vi "AttackerStop.vi"(6 "atacando contra?":bool, 7 "AI Parameters":T1={"GotoKick"={"Dist do cone a frente"=150.0, "attacker farback"=1500.0, "Perto"=300.0, "Dist a frente da bola"=0.0, "min dist to kick"=150.0, "Constante do Renault"=0.05, "distance between ball and robot"=200.0, "Time Target \nto transition"=0.3}, "Attacker"={"CC chute"=0.09, "CC passe"=0.045, "Kick Force"=100.0}, "Defender"={"D max"=1700.0, "Velocidade p/ o robô avançar"=1000.0, "Kick Force"=100.0}, "Timeout"={"Field/v in x"=6, "Dist Robots"=300, "Dist up in y"=300}, "Pose Striker"={"dist"=200.0, "Numeric"=-4.0, "dist 2"=200.0}, "Dist Stop"=300.0, "Distance when ball out"=200, "Defence central gap "=150.0} {"Defence central gap" format="%#_13g"; "Dist Stop" format="%#_13g"; "Pose Striker"."Numeric" format="%#_13g"; "Defender"."Kick Force" format="%#_13g"; "Defender"."Velocidade p/ o robô avançar" format="%#_13g"; "Attacker"."Kick Force" format="%#_13g"; "Attacker"."CC passe" format="%#_13g"; "Attacker"."CC chute" format="%#_13g"; "GotoKick"."distance between ball and robot" format="%#_13g"; "GotoKick"."min dist to kick" format="%#_13g"; "GotoKick"."Dist a frente da bola" format="%#_13g"; "GotoKick"."Perto" format="%#_13g"; "GotoKick"."attacker farback" format="%#_13g"; "GotoKick"."Dist do cone a frente" format="%#_13g"}, 8 "IA State Input 2":T2, 9 "balls":T6[](array[typedef]), 10 "Field Size in":T7, 11 "Robot in":T3={"id"=0, "function"=enum."Attacker", "x"=0.0, "y"=0.0, "orientation"=0.0, "v_tangent"=0.0, "v_normal"=0.0, "v_ang"=0.0, "kick_x"=0.0, "kick_z"=0.0, "dribble"=FALSE, "Timestamp"=timestamp(0 s since 1904-01-01), "dest_x"=0.0, "dest_y"=0.0, "dest_orientation"=0.0, "estimatives"={"est_v_tangent"=0.0, "est_v_normal"=0.0, "est_vx"=0.0, "est_vy"=0.0, "Pos Robot Est"=[]}, "dest_x_kick"=0.0, "dest_y_kick"=0.0, "Gap Coord"=[], "States"=enum."GoToTangent"}) -> (3 "Robot out":T3={"id"=0, "function"=enum."Attacker", "x"=0.0, "y"=0.0, "orientation"=0.0, "v_tangent"=0.0, "v_normal"=0.0, "v_ang"=0.0, "kick_x"=0.0, "kick_z"=0.0, "dribble"=FALSE, "Timestamp"=timestamp(0 s since 1904-01-01), "dest_x"=0.0, "dest_y"=0.0, "dest_orientation"=0.0, "estimatives"={"est_v_tangent"=0.0, "est_v_normal"=0.0, "est_vx"=0.0, "est_vy"=0.0, "Pos Robot Est"=[]}, "dest_x_kick"=0.0, "dest_y_kick"=0.0, "Gap Coord"=[], "States"=enum."GoToTangent"})   [LabVIEW 2016]
uses:
  Core/Field Size.ctl
  Core/AI Robot.ctl
  Functions Enum.ctl
  AttackerStates.ctl
  Core/AI Ball.ctl
  Core/AI Input.ctl
  Core/AI Judge.ctl
  Command Enum.ctl
  Util/Events/Events.ctl
  AI Parameters.ctl
  <vilib>/Analysis/_algsub.llb/Real Vector Norm.vi
  <vilib>/Analysis/NI_AALPro.lvlib
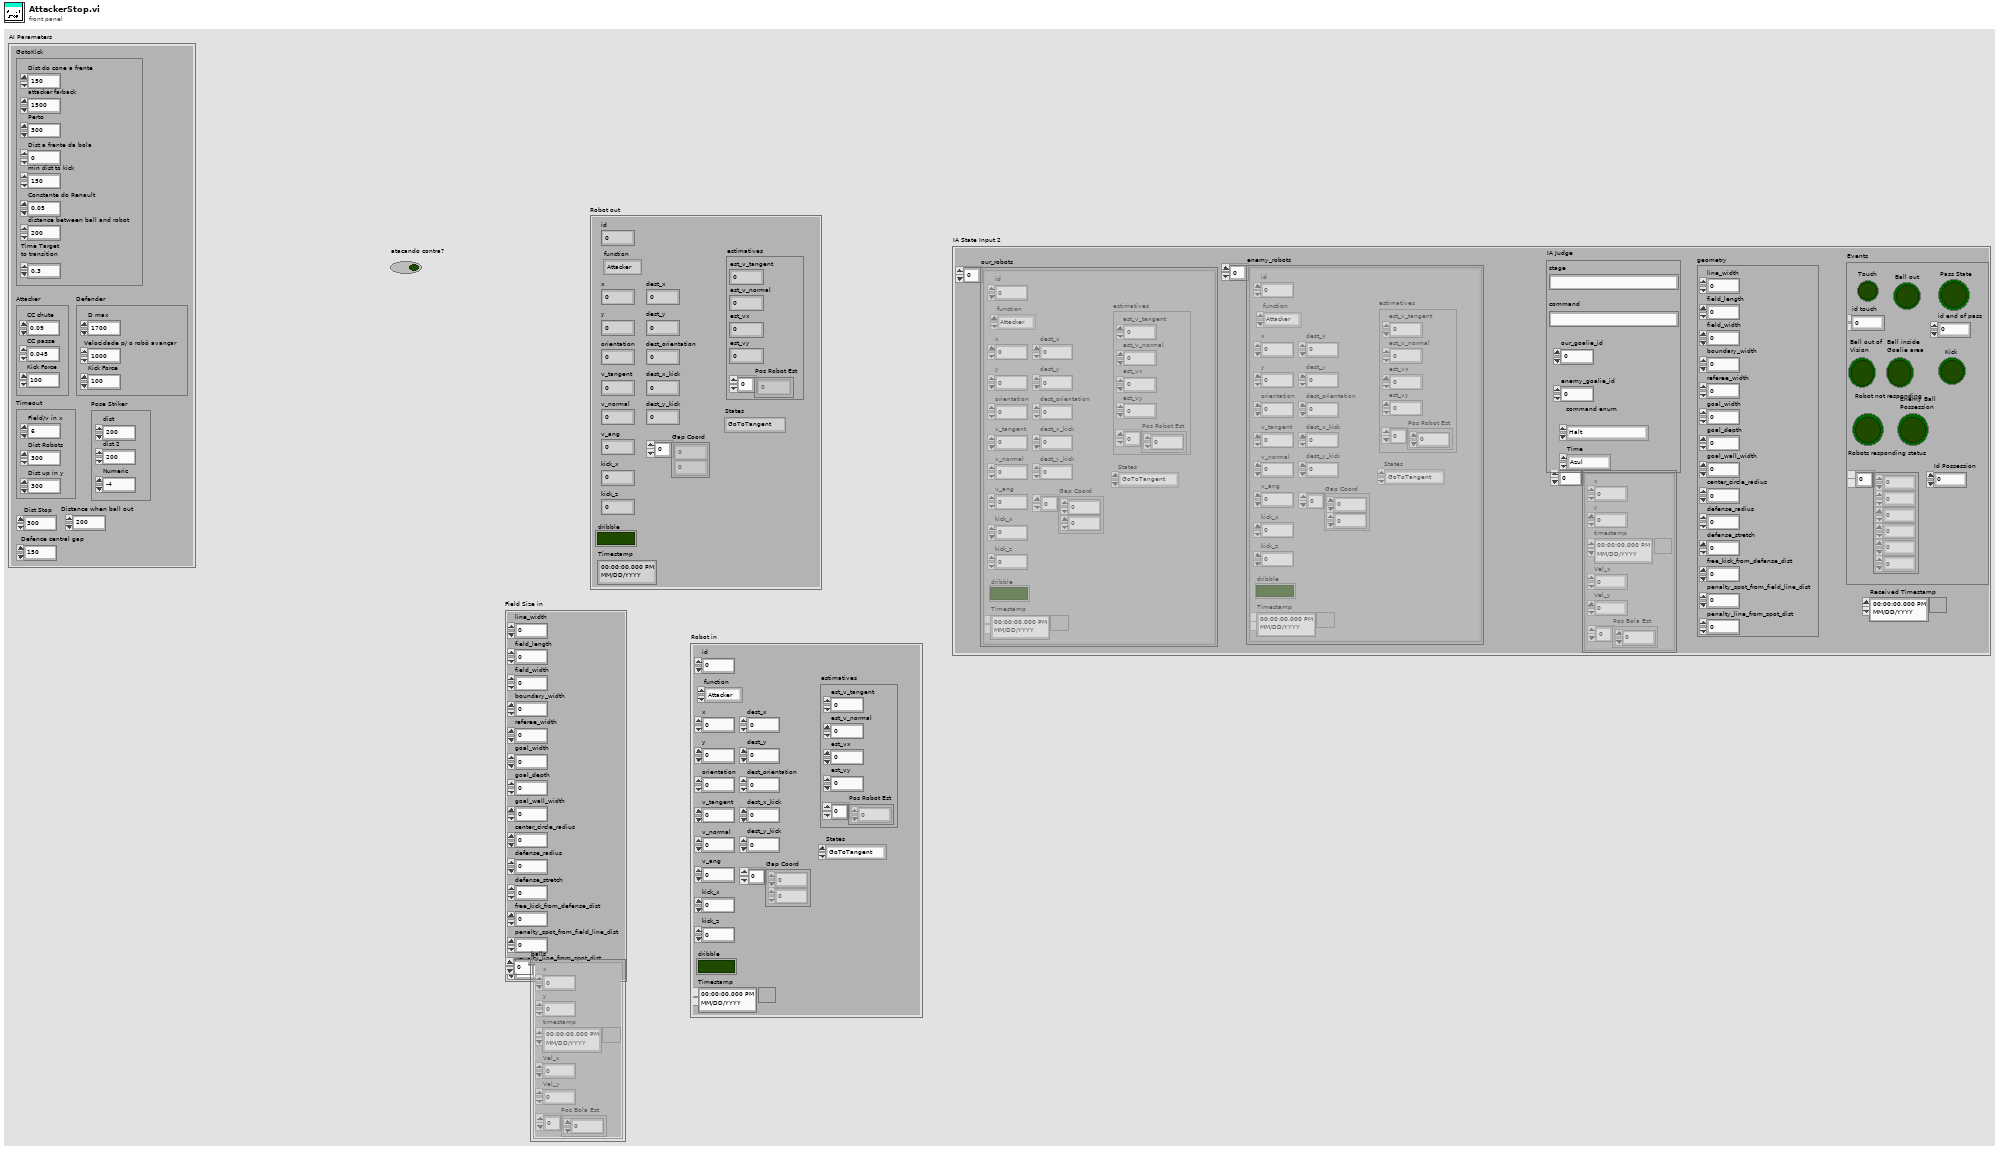
[diagram p1: front panel]
types:
  T1 = typedef "AI Parameters.ctl" = cluster{"GotoKick":cluster{"Dist do cone a frente":dbl, "attacker farback":dbl, "Perto":dbl, "Dist a frente da bola":dbl, "min dist to kick":dbl, "Constante do Renault":dbl, "distance between ball and robot":dbl, "Time Target \nto transition":dbl}, "Attacker":cluster{"CC chute":dbl, "CC passe":dbl, "Kick Force":dbl}, "Defender":cluster{"D max":dbl, "Velocidade p/ o robô avançar":dbl, "Kick Force":dbl}, "Timeout":cluster{"Field/v in x":u32, "Dist Robots":u32, "Dist up in y":u32}, "Pose Striker":cluster{"dist":dbl, "Numeric":dbl, "dist 2":dbl}, "Dist Stop":dbl, "Distance when ball out":i32, "Defence central gap ":dbl}
  T2 = typedef "AI Input.ctl" = cluster{"our_robots":T3[], "enemy_robots":T3[], "balls":T6[], "geometry":T7, "IA Judge":T8, "Received Timestamp":timestamp, "Events":T10}
  T3 = typedef "AI Robot.ctl" = cluster{"id":u32, "function":T4, "x":dbl, "y":dbl, "orientation":dbl, "v_tangent":dbl, "v_normal":dbl, "v_ang":dbl, "kick_x":dbl, "kick_z":dbl, "dribble":bool, "Timestamp":timestamp, "dest_x":dbl, "dest_y":dbl, "dest_orientation":dbl, "estimatives":cluster{"est_v_tangent":dbl, "est_v_normal":dbl, "est_vx":dbl, "est_vy":dbl, "Pos Robot Est":dbl[]}, "dest_x_kick":dbl, "dest_y_kick":dbl, "Gap Coord":dbl[], "States":T5}
  T4 = typedef "Functions Enum.ctl" = enum16{"Attacker", "Goalie", "Defender", "Striker", "Goto 0", "Dummy", "Kicker", "ZigZag"}
  T5 = typedef "AttackerStates.ctl" = enum16{"Pass", "GoToTangent", "BallGetting", "GoToKick", ""}
  T6 = typedef "AI Ball.ctl" = cluster{"x":dbl, "y":dbl, "timestamp":timestamp, "Vel_x":dbl, "Vel_y":dbl, "Pos Bola Est":dbl[]}
  T7 = typedef "Field Size.ctl" = cluster{"line_width":u32, "field_length":u32, "field_width":u32, "boundary_width":u32, "referee_width":u32, "goal_width":u32, "goal_depth":u32, "goal_wall_width":u32, "center_circle_radius":u32, "defense_radius":u32, "defense_stretch":u32, "free_kick_from_defense_dist":u32, "penalty_spot_from_field_line_dist":u32, "penalty_line_from_spot_dist":u32}
  T8 = typedef "AI Judge.ctl" = cluster{"stage":string, "command":string, "our_goalie_id":dbl, "enemy_goalie_id":dbl, "command enum":T9, "Time":enum16{"Azul", "Amarelo"}}
  T9 = typedef "Command Enum.ctl" = enum16{"Halt", "Stop", "Force Start", "PKA Normal Start", "Prepare Kickoff Ally", "PKE Normal Start", "Prepare Kickoff Enemy", "Prepare Penalty Ally", "PPA Normal Start", "Prepare Penalty Enemy", "PPE Normal Start", "Direct Free Enemy", "Direct Free Ally", "Indirect Free Enemy", "Indirect Free Ally", "Timeout Enemy", "Timeout Ally", "Goal Enemy", "Goal Ally", "Ball Placement Enemy", "Ball Placement Ally", "Normal Half Time", "Extra Time Break", "Extra Half Time", "None"}
  T10 = typedef "Events.ctl" = cluster{"Touch":bool, "Ball out":bool, "id touch":dbl, "Ball out of \nVision":bool, "Ball inside \nGoalie area":bool, "Robot not responding":bool, "Robots responding status":dbl[], "Enemy Ball \nPossession":bool, "Pass State":bool, "id end of pass":dbl, "Kick":bool, "Id Possession":dbl}
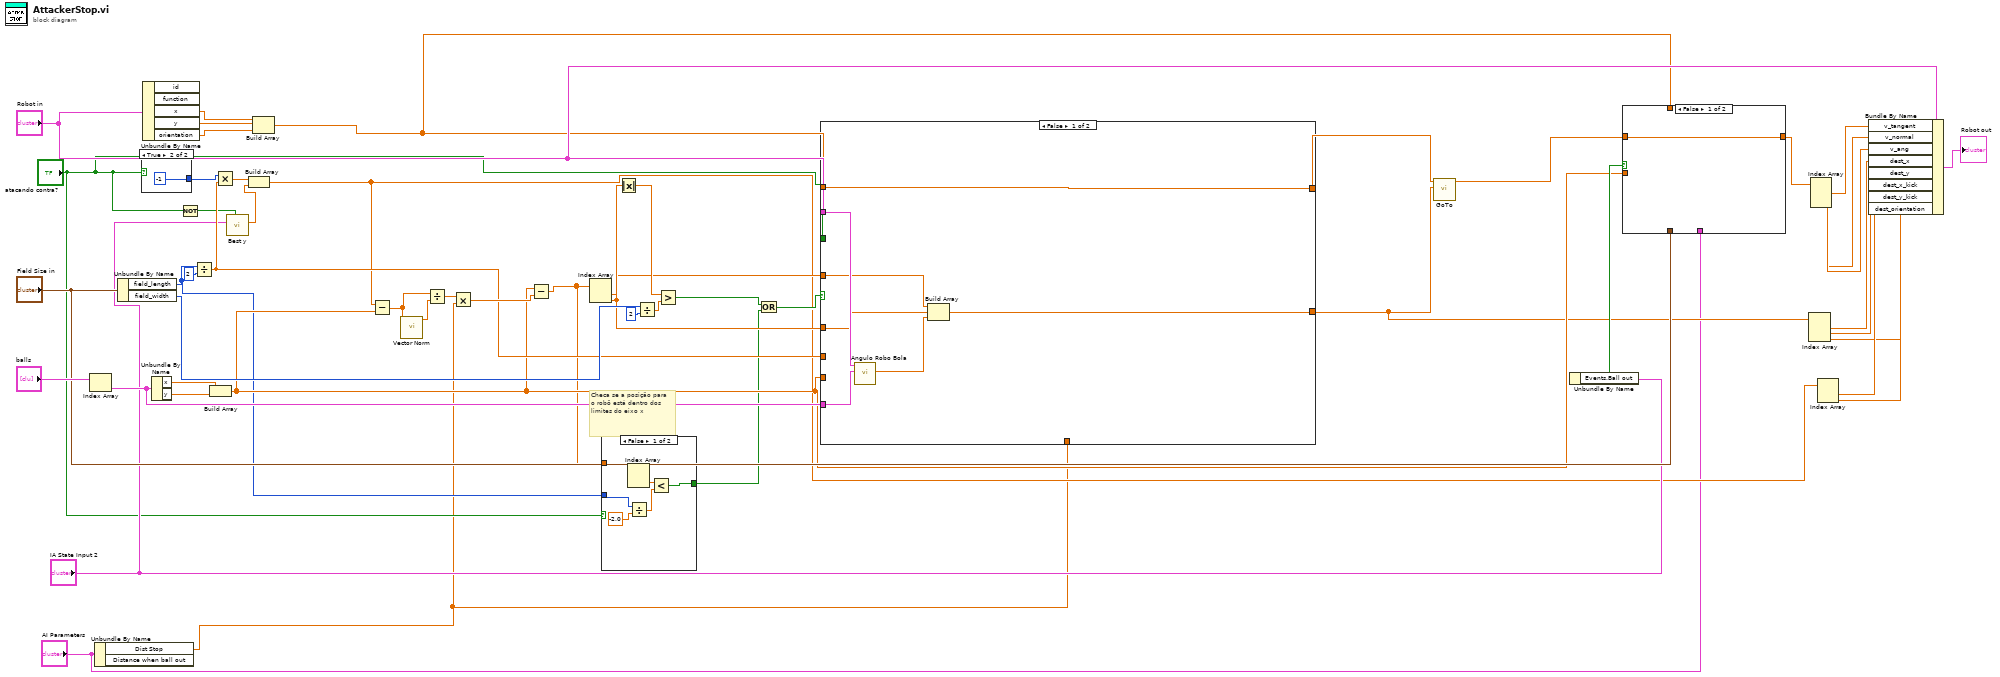
[diagram p0: block diagram]
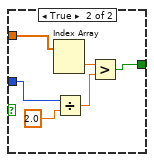
[diagram p2: hidden frame]
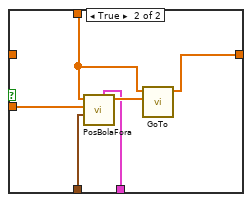
[diagram p3: hidden frame]
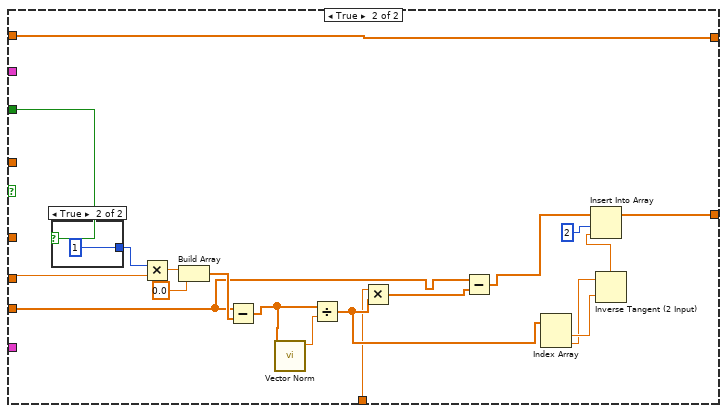
[diagram p4: hidden frame]
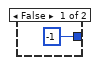
[diagram p5: hidden frame]
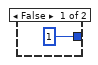
[diagram p6: hidden frame]
diagram:
  # "Checa se a posição para o robõ está dentro dos limites do eixo x"
  n1 = Index Array(array="balls") -> (element=w38:T6)  [unwired: 1 in]
  n2 = Unbundle By Name("AI Parameters") -> ("Dist Stop"=w2:dbl)  [unwired: 1 out]
  n3 = Unbundle By Name("Field Size in") -> ("field_length"=w16:u32, "field_width"=w40:u32)
  n4 = case shown="True" "atacando contra?" {
    tunnel: [1 -1] -> w49
    frame False {
    }
    frame True {
    }
  }
  n5 = Unbundle By Name("Robot in") -> ("x"=w35:dbl, "y"=w34:dbl, "orientation"=w33:dbl)  [unwired: 2 out]
  n6 = Unbundle By Name(w38) -> ("x"=w48:dbl, "y"=w47:dbl)
  n7 = Not(x="atacando contra?") -> (.not. x?=w8:bool)
  n8 = Divide(x=w16, y=u32 2) -> (x/y=w19:dbl)
  n9 = Build Array(w48, w47) -> (w18:dbl[])
  n10 = Multiply(x=w49, y=w19) -> (x*y=w46:dbl)
  n11 = call "Best y.vi"("inimigos"=w8, "IA State"="IA State Input 2") -> ("Best y"=w9:dbl)  [unwired: 6 in, 3 out]
  n12 = Build Array(w46, w9) -> (w6:dbl[])
  n13 = Build Array(w35, w34, w33) -> (w24:dbl[])
  n14 = Subtract(x=w6, y=w18) -> (x-y=w45:dbl[])
  n15 = call-poly <vilib>:"Vector Norm.vi"("Input Vector"=w45) -> ("norm"=w44:dbl)  [unwired: 9 in, 1 out]
  n16 = Divide(x=w45, y=w44) -> (x/y=w43:dbl[])
  n17 = Multiply(x=w43, y=w2) -> (x*y=w22:dbl[])
  n18 = Subtract(x=w18, y=w22) -> (x-y=w17:dbl[])
  n19 = Index Array(array=w17) -> (element #1=w36:dbl, element #2=w37:dbl)  [unwired: 2 in]
  n20 = case shown="False" "atacando contra?" {
    tunnel: w16 -> [w57 w63]
    tunnel: [w56 w60] -> w11
    tunnel: w17 -> [w55 w64]
    frame False {
      n21 = Index Array(array=w55) -> (element #1=w59:dbl)  [unwired: 2 in, 1 out]
      n22 = Divide(x=w57, y=-2.0) -> (x/y=w58:dbl)
      n23 = Less?(x=w59, y=w58) -> (x < y?=w56:bool)
    }
    frame True {
      n24 = Index Array(array=w64) -> (element #1=w62:dbl)  [unwired: 2 in, 1 out]
      n25 = Divide(x=w63, y=2.0) -> (x/y=w61:dbl)
      n26 = Greater?(x=w62, y=w61) -> (0:w60:bool)
    }
  }
  n27 = Absolute Value(x=w37) -> (abs(x)=w42:dbl)
  n28 = Divide(x=w40, y=u32 2) -> (x/y=w39:dbl)
  n29 = Greater?(x=w42, y=w39) -> (0:w12:bool)
  n30 = Or(x=w12, y=w11) -> (x .or. y?=w13:bool)
  n31 = case shown="False" w13 {
    tunnel: w38 -> [w72 _]
    tunnel: "Robot in" -> [w71 _]
    tunnel: w37 -> [w69 _]
    tunnel: w36 -> [w68 _]
    tunnel: w24 -> [w67 w78]
    tunnel: w18 -> [_ w75]
    tunnel: "atacando contra?" -> [_ w85]
    tunnel: w19 -> [_ w90]
    tunnel: [w67 w78] -> w15
    tunnel: [w66 w77] -> w14
    tunnel: w2 -> [_ w73]
    frame False {
      n32 = call "Angulo Robo Bola.vi"("Ball"=w72, "Robot"=w71) -> ("Angulo"=w70:dbl)  [unwired: 9 in]
      n33 = Build Array(w68, w69, w70) -> (w66:dbl[])
    }
    frame True {
      n34 = case shown="True" w85 {
        tunnel: [-1 1] -> w91
        frame False {
        }
        frame True {
        }
      }
      n35 = Multiply(x=w91, y=w90) -> (x*y=w89:dbl)
      n36 = Build Array(w89, 0.0 ("element")) -> (w84:dbl[])
      n37 = Subtract(x=w75, y=w84) -> (x-y=w86:dbl[])
      n38 = call-poly <vilib>:"Vector Norm.vi"("Input Vector"=w86) -> ("norm"=w87:dbl)  [unwired: 9 in, 1 out]
      n39 = Divide(x=w86, y=w87) -> (x/y=w79:dbl[])
      n40 = Multiply(x=w73, y=w79) -> (x*y=w76:dbl[])
      n41 = Subtract(x=w75, y=w76) -> (x-y=w74:dbl[])
      n42 = Index Array(array=w79) -> (element #1=w81:dbl, element #2=w80:dbl)  [unwired: 2 in]
      n43 = Inverse Tangent (2 Input)(1:w81, 2:w80) -> (0:w82:dbl)
      n44 = Insert Into Array(array=w74, index=2, new element=w82) -> (w77:dbl[])
    }
  }
  n45 = call "GoTo.vi"("Target"=w14, "Position"=w15) -> ("Output\nVelocity"=w23:dbl[])  [unwired: 8 in, 1 out]
  n46 = Unbundle By Name("IA State Input 2") -> ("Events.Ball out"=w32:bool)
  n47 = case shown="False" w32 {
    tunnel: w23 -> [w94 _]
    tunnel: [w94 w96] -> w26
    tunnel: "Field Size in" -> [_ w100]
    tunnel: w24 -> [_ w97]
    tunnel: w18 -> [_ w99]
    tunnel: "AI Parameters" -> [_ w95]
    frame False {
    }
    frame True {
      n48 = call "PosBolaFora.vi"("AI Parameters"=w95, "Field Size in"=w100, "Position da bola"=w99, "Position do robot"=w97) -> ("Target"=w98:dbl[])  [unwired: 7 in]
      n49 = call "GoTo.vi"("Target"=w98, "Position"=w97) -> ("Output\nVelocity"=w96:dbl[])  [unwired: 8 in, 1 out]
    }
  }
  n50 = Index Array(array=w14) -> (element #1=w21:dbl, element #2=w20:dbl, element #3=w3:dbl)  [unwired: 3 in]
  n51 = Index Array(array=w26) -> (element #1=w29:dbl, element #2=w30:dbl, element #3=w31:dbl)  [unwired: 3 in]
  n52 = Index Array(array=w6) -> (element #1=w5:dbl, element #2=w4:dbl)  [unwired: 2 in]
  n53 = Bundle By Name(cluster="Robot in", "v_tangent"=w29, "v_normal"=w30, "v_ang"=w31, "dest_x"=w21, "dest_y"=w20, "dest_x_kick"=w5, "dest_y_kick"=w4, "dest_orientation"=w3) -> (→"Robot out":T3)
